vi "recover.vi"(8 "error in (no error)":errorcluster, 11 "Camera Handle":u32=16842752) -> (0 "error out":errorcluster, 2 "Temperature":dbl=-75.0, 3 "Camera Handle":u32=16842752)   [LabVIEW 2015]
uses:
  LabVIEW/Examples2014_6_0_2_9/Fast Examples/Open-Close Hardware/CamHandle.vi
panel:
  out "Pixel Time":i32=500
  in  "Bypass Cooling":bool
  out "Frame Rate":dbl=1203.5142616440007
  out "Vertical Index":u32
  out "Custom Chip Enabled":bool
  out "Vertical Timing":dbl=3.2
  out "Readout Time":dbl=0.8308999999999999
  out "Bit Depth":i32=16
  out "ReadOut Port":i32=2
  out "ADC Offset":i32=-1
  out "ADC Gain":i32=3
  out "ADC Speed":i32=2000
  in  "Error Code(s)":string="Ready"
  in  "Write Tab Control":T1(tab)=enum."ROI"
  in  "Frames to collect (nframe)":u32=1 min=1 step=1
  in  "Exposure":dbl min=0.0 step=0.001 format="%.3f"
  in  "Timing Mode":u32(ring)=3 items=["Free Run/Timed"=1, "External Sync"=3, "Shift per Trigger"=13]
  in  "Trigger Edge":u32(ring)=2 items=["Positive Edge"=1, "Negative Edge"=2]
  in  "Collection Mode":u32(ring)=1 items=["Focus"=1, "N-Frame"=2, "Asynchronous"=3]
  in  "Readut Mode":u16(ring)=1 items=["Full Frame"=1, "Kinetics"=10]
  in  "Temperature 2":dbl=-75.0 format="%.2f"
  in  "Speed":i32=-2 min=-3 step=1
  in  "Gain":i32(ring)=3 items=["Don't Change "=-1, "Low"=1, "Medium"=2, "High"=3]
  in  "Offset":i32=-1 min=-1 step=1
  in  "Readout Port":i32(ring)=2 items=["Don't Change"=-1, "Low Noise"=1, "High capacity"=2]
  in  "Open":u32
  in  "Close":u32
  in  "Shutter State":u16(ring)=3 items=["Always Closed"=1, "Open Each Exposure"=2, "Open at Begining of Acquisition"=3, "Open While Waiting for Trigger"=4]
  in  "Minium Block Size":u32=1
  in  "Number of Minimum Blocks":u32=1
  in  "Number of Clean/Clears cycles":u32
  in  "Number of Strips per Clean":u32=100
  in  "Continous Cleans":bool
  in  "Skip Serial Register Clean":bool=TRUE
  in  "Kinetics Window Height":u32
  in  "Active Y Size":u32=100
  in  "Post Y":u32=8
  in  "Pre Y":u32=8
  in  "Active X Size":u32=1340
  in  "Post X":u32
  in  "Pre X":u32
  in  "Vertical Timing Index":u32
  in  "Enable  Custom Chip":bool
  in  "Logic Output":u16(ring)=3 items=["Not Scan / Not Reading"=1, "Shutter Open"=2, "Not Ready/Busy"=3, "Always Low"=4, "Always High"=8]
  in  "Invert":bool
  out "Y Size ROI":u32=50
  out "X Size ROI":u32=1340
  in  "Y Bin":u32=100 min=1 step=1
  in  "Y End":u32=100 min=1 step=1
  in  "Y Start":u32=1 min=1 step=1
  in  "X Bin":u32=1 min=1 step=1
  in  "X End":u32=1340 min=1 max=100000 step=1
  in  "X Start":u32=1 min=1 step=1
  in  "Camera Number":u32=1
  in  "INI Flag":bool=TRUE
  # "Triggering"
  # "Seconds"
  # "Temperature"
  # "°C"
  # "ADC"
  # "-3 = Slowest speed\n-2 = Fastest speed\n-1 =Default speed or enter speed in kHz"
  # "Shutter"
  # "Shutter Times"
  # "ms"
  # "Cleans / Clears"
  # "Custom Chip and Timing"
  # "Kinetics Timing"
  # "Logic Output"
  # "Region Of Interest"
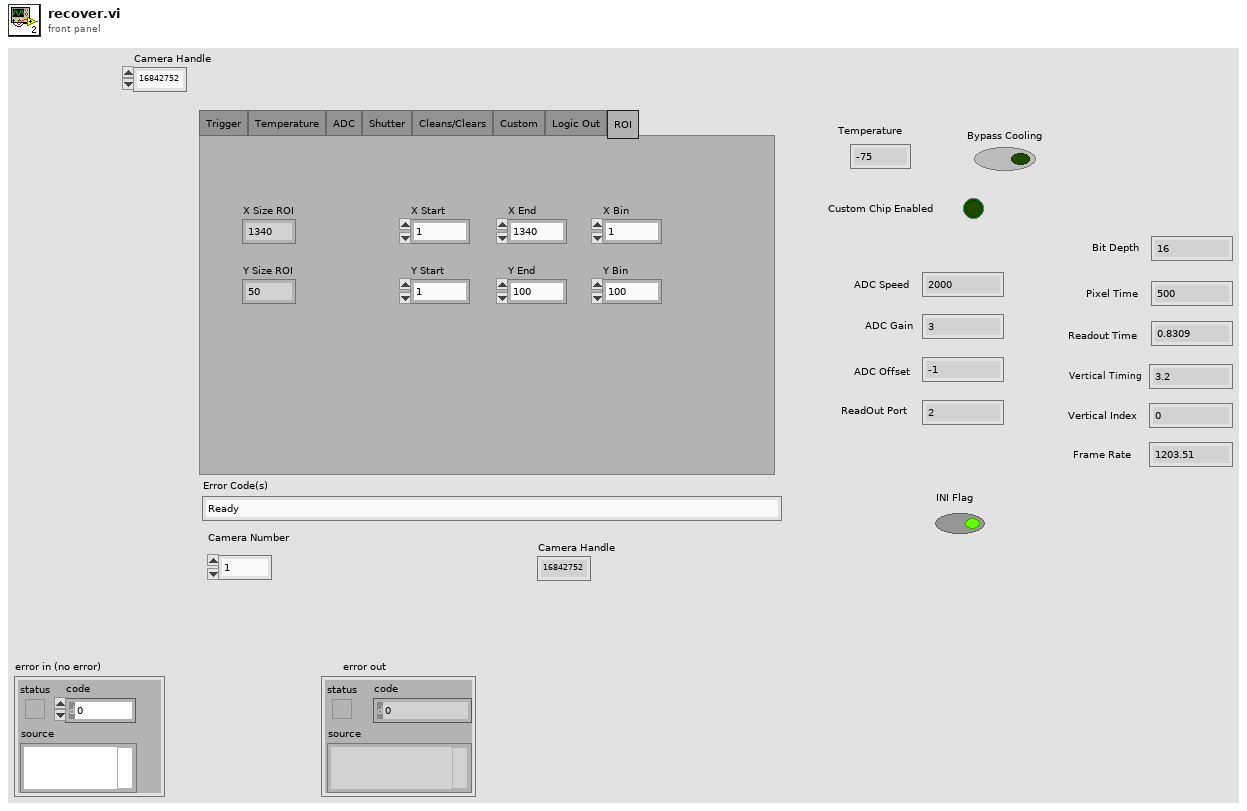
[diagram p1: front panel]
types:
  T1 = enum32{"Trigger", "Temperature", "ADC", "Shutter", "Cleans/Clears", "Custom", "Logic Out", "ROI"}
  T2 = cluster{"Camera Number":i32, "ROI Number":i32, "X Start":i32, "X End":i32, "X Bin":i32, "Y Start":i32, "Y End":i32, "Y Bin":i32}
  T3 = cluster{"Pre Y":u32, "Post Y":u32, "Active Y":u32, "Pre X":u32, "Post X":u32, "Active X":u32, "Custom Chip Enabled":bool, "Vertical Timing Index":u32}
  T4 = cluster{"Exposure":dbl, "Collection Mode":u32, "Timing Mode":u32, "Trigger Edge":u32, "Temperature":dbl}
  T5 = cluster{"ADC Speed":i32, "ADC Gain":i32, "ADC Offset":i32, "Readout Port":i32, "Num Cleans":u32, "Num Strips per Clean":u32, "Mini Block Size":u32, "Num Min Blocks":u32, "Continous Cleans":bool, "Skip Serial Reg Clean":bool}
  T6 = cluster{"Shutter State":u16, "Open Comp Time ":u32, "Close Comp Time":u32, "Logic Out Setting":u32, "Logic Out Invert":bool}
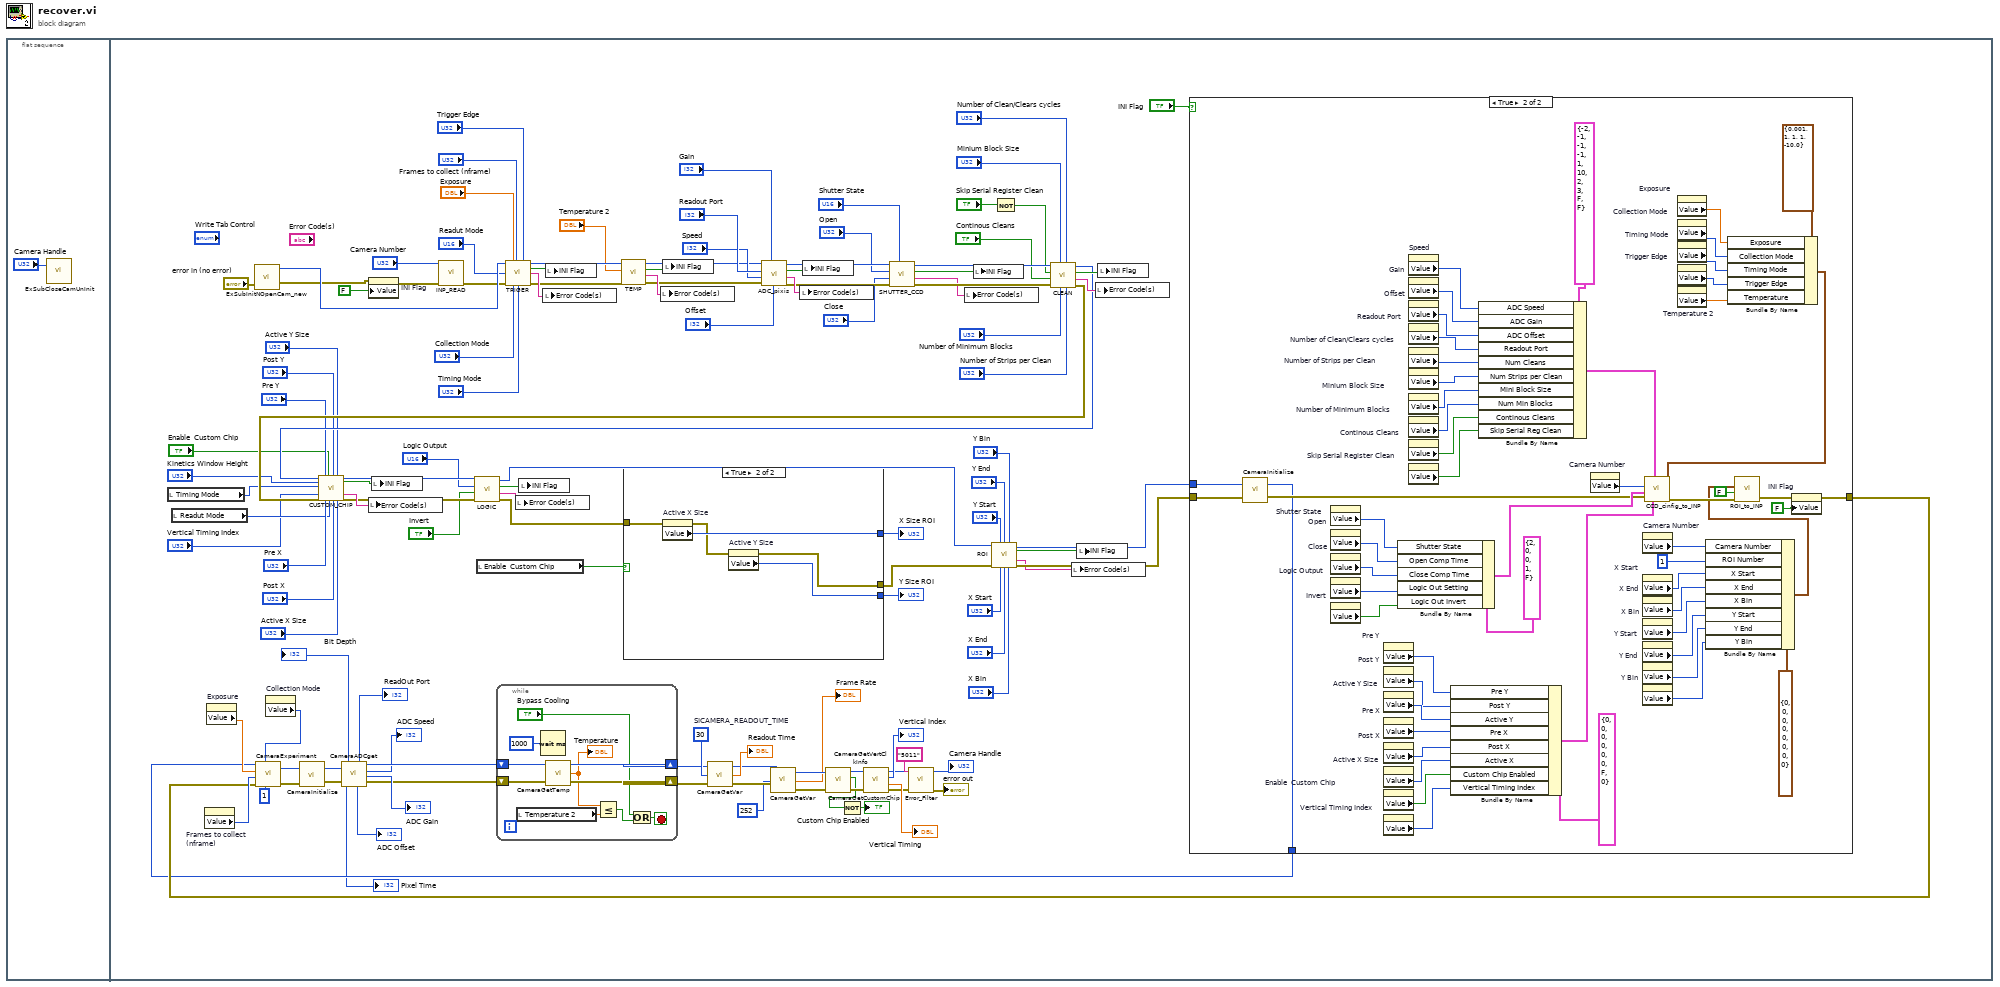
[diagram p0: block diagram]
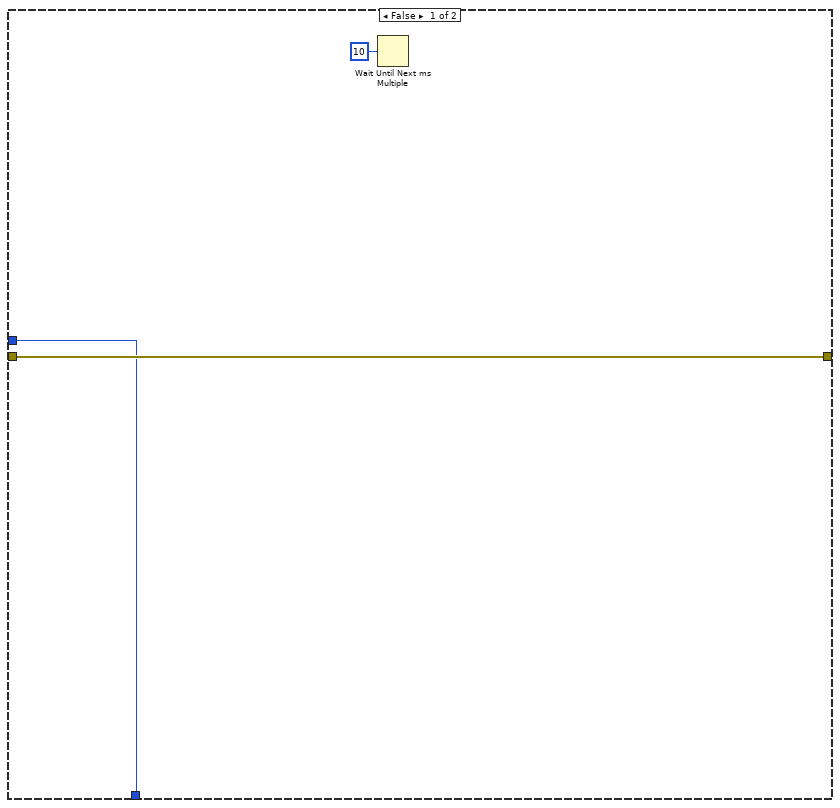
[diagram p2: hidden frame]
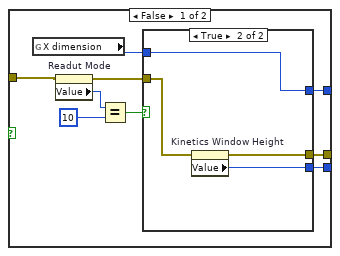
[diagram p3: hidden frame]
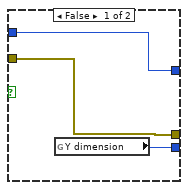
[diagram p4: hidden frame]
diagram:
  n1 = flat-sequence {
    frame #0 {
      n2 = call "ExSubCloseCamUnInit.vi"("Camera Handle"="Camera Handle") -> ()  [unwired: 1 in, 1 out]
    }
    frame #1 {
      w40 = 30  # SICAMERA_READOUT_TIME
      n3 = local read "Timing Mode"() -> (w69:u32)
      n4 = local read "Readut Mode"() -> (w70:u16)
      n5 = property on="Frames to collect (nframe)" class="DigNum (strict)"() -> ("Value"=w19:u32)  [unwired: 2 in, 2 out]
      n6 = property on="Exposure" class="DigNum (strict)"() -> ("Value"=w22:dbl)  [unwired: 2 in, 2 out]
      n7 = call "ExSubInitNOpenCam_new.vi"("error in (no error)"="error in (no error)") -> ("Camera Handle"=w121:u32, "error out"=w6:errorcluster)  [unwired: 1 out]
      n8 = property on="Collection Mode" class="Ring (strict)"() -> ("Value"=w17:u32)  [unwired: 2 in, 2 out]
      n9 = property on="INI Flag" class="Bool (strict)"(error in=w6, "Value"=FALSE) -> (error out=w106:errorcluster)  [unwired: 1 in, 1 out]
      n10 = call "INP_READ.vi"("error in (no error)"=w106, "Camera Number"="Camera Number") -> ("error out"=w105:errorcluster)  [unwired: 4 in, 5 out]
      n11 = local read "Enable  Custom Chip"() -> (w60:bool)
      n12 = call "TRIGER.vi"("Camera Handle"=w121, "Exposure (sec)"="Exposure", "Number of frams"="Frames to collect (nframe)", "Trigger Edge"="Trigger Edge", "ReadOut Mode"="Readut Mode", "error out"=w105, "Acquire / Focus Flag"="Collection Mode", "Timing Mode"="Timing Mode") -> ("Camera Handle"=w112:u32, "INI Flag"=w114:bool, "String"=w113:string, "error out"=w111:errorcluster)  [unwired: 4 in]
      n13 = local write "Error Code(s)"(w113) -> ()
      n14 = local write "INI Flag"(w114) -> ()
      n15 = call "TEMP.vi"("error in (no error)"=w111, "Temperature"="Temperature 2", "Camera Handle"=w112) -> ("error out"=w102:errorcluster, "String"=w109:string, "INI Flag"=w108:bool, "Camera Handle"=w97:u32)  [unwired: 5 in]
      n16 = local write "Error Code(s)"(w109) -> ()
      n17 = local write "INI Flag"(w108) -> ()
      n18 = call "ADC_pixis.vi"("ADC offset"="Offset", "ADC Gain"="Gain", "error in (no error)"=w102, "ADC Speed"="Speed", "Read Out port"="Readout Port", "Camera Handle"=w97) -> ("error out"=w95:errorcluster, "string"=w98:string, "INI Flag"=w99:bool, "Camera Handle"=w96:u32)  [unwired: 2 in]
      n19 = local write "Error Code(s)"(w98) -> ()
      n20 = local write "INI Flag"(w99) -> ()
      n21 = call "SHUTTER_CCD.vi"("Shutter State"="Shutter State", "error out"=w95, "Shutter Comp Time: Pre Open"="Close", "Shutter Comp Time: Post Open"="Open", "Camera Handle"=w96) -> ("error out"=w90:errorcluster, "String"=w89:string, "INI Flag"=w88:bool, "Camera Handle"=w91:u32)  [unwired: 3 in]
      n22 = local write "Error Code(s)"(w89) -> ()
      n23 = local write "INI Flag"(w88) -> ()
      n24 = Not(x="Skip Serial Register Clean") -> (.not. x?=w11:bool)
      n25 = call "CLEAN.vi"("Number of Strips Per Clear"="Number of Strips per Clean", "Number of Clears"="Number of Clean/Clears cycles", "Number of Minimum blocks"="Number of Minimum Blocks", "Minimum Block Size"="Minium Block Size", "error out"=w90, "Continous Clean"="Continous Cleans", "Skip Serial Reg Clean"=w11, "Camera Handle"=w91) -> ("error out 2"=w79:errorcluster, "String"=w82:string, "INI Flag"=w81:bool, "CameraHandle"=w80:u32)
      n26 = call "CUSTOM_CHIP.vi"("Camera Handle"=w80, "Window Size"="Kinetics Window Height", "TriggerMode"=w69, "Vertical Clock"="Vertical Timing Index", "error out"=w79, "Pre Y"="Pre Y", "Pre X"="Pre X", "Enable / Disable Custom Chip"="Enable  Custom Chip", "ReadOut Mode"=w70, "Post Y"="Post Y", "Post X"="Post X", "Parallel (Y) Size"="Active Y Size", "Serial (X) Size"="Active X Size") -> ("Camera Handle"=w66:u32, "INI Flag"=w72:bool, "String"=w71:string, "error out"=w65:errorcluster)  [unwired: 3 in]
      n27 = local write "Error Code(s)"(w71) -> ()
      n28 = local write "INI Flag"(w72) -> ()
      n29 = call "LOGIC.vi"("error out"=w65, "Invert"="Invert", "Logic Output"="Logic Output", "Camera Handle"=w66) -> ("error out 2"=w59:errorcluster, "String"=w61:string, "INI Flag"=w62:bool, "Camera Handle"=w58:u32)  [unwired: 4 in]
      n30 = local write "Error Code(s)"(w61) -> ()
      n31 = local write "INI Flag"(w62) -> ()
      n32 = case shown="True" w60 {
        tunnel: [w197 w213] -> w49
        tunnel: [w196 w212] -> w50
        tunnel: w59 -> [w194 w210]
        tunnel: [w195 w209] -> w57
        frame False {
          n33 = global read "CamHandle.vi" "X dimension"() -> (w198:u32)
          n34 = property on="Readut Mode" class="Ring (strict)"(error in=w194) -> (error out=w193:errorcluster, "Value"=w199:u16)  [unwired: 1 in, 1 out]
          n35 = Equal?(x=w199, y=10) -> (x = y?=w200:bool)
          n36 = case shown="True" w200 {
            tunnel: w198 -> [w204 w208]
            tunnel: [w204 w208] -> w197
            tunnel: [w203 w207] -> w196
            tunnel: [w202 w206] -> w195
            tunnel: w193 -> [w202 w205]
            frame False {
              n37 = global read "CamHandle.vi" "Y dimension"() -> (w203:u32)
            }
            frame True {
              n38 = property on="Kinetics Window Height" class="DigNum (strict)"(error in=w205) -> (error out=w206:errorcluster, "Value"=w207:u32)  [unwired: 1 in, 1 out]
            }
          }
        }
        frame True {
          n39 = property on="Active X Size" class="DigNum (strict)"(error in=w210) -> (error out=w211:errorcluster, "Value"=w213:u32)  [unwired: 1 in, 1 out]
          n40 = property on="Active Y Size" class="DigNum (strict)"(error in=w211) -> (error out=w209:errorcluster, "Value"=w212:u32)  [unwired: 1 in, 1 out]
        }
      }
      "X Size ROI" <- w49
      "Y Size ROI" <- w50
      n41 = call "ROI.vi"("Camera Handle"=w58, "Y Start"="Y Start", "Y End"="Y End", "Y Bin"="Y Bin", "error in"=w57, "X Start"="X Start", "X End"="X End", "X Bin"="X Bin") -> ("Camera Handle"=w16:u32, "INI Flag"=w48:bool, "String"=w7:string, "error out"=w15:errorcluster)  [unwired: 4 in]
      n42 = local write "Error Code(s)"(w7) -> ()
      n43 = local write "INI Flag"(w48) -> ()
      n44 = local write "Error Code(s)"(w82) -> ()
      n45 = local write "INI Flag"(w81) -> ()
      n46 = case shown="True" "INI Flag" {
        tunnel: w15 -> [w136 w164]
        tunnel: [w136 w162] -> w5
        tunnel: w16 -> [w134 w138]
        tunnel: [w134 w137] -> w4
        frame False {
          n47 = Wait Until Next ms Multiple(millisecond multiple=u32 10) -> ()  [unwired: 1 out]
        }
        frame True {
          n48 = call <userlib>:"CameraInitialize.vi"("error in"=w164, "Camera Handle"=w138) -> ("error out"=w165:errorcluster, "Camera Handle"=w137:u32)
          n49 = property on="Shutter State" class="Ring (strict)"() -> ("Value"=w186:u16)  [unwired: 2 in, 2 out]
          n50 = property on="Open" class="DigNum (strict)"() -> ("Value"=w187:u32)  [unwired: 2 in, 2 out]
          n51 = property on="Close" class="DigNum (strict)"() -> ("Value"=w188:u32)  [unwired: 2 in, 2 out]
          n52 = property on="Logic Output" class="Ring (strict)"() -> ("Value"=w189:u16)  [unwired: 2 in, 2 out]
          n53 = property on="Invert" class="Bool (strict)"() -> ("Value"=w190:bool)  [unwired: 2 in, 2 out]
          n54 = property on="Pre Y" class="DigNum (strict)"() -> ("Value"=w159:u32)  [unwired: 2 in, 2 out]
          n55 = property on="Post Y" class="DigNum (strict)"() -> ("Value"=w151:u32)  [unwired: 2 in, 2 out]
          n56 = property on="Active Y Size" class="DigNum (strict)"() -> ("Value"=w154:u32)  [unwired: 2 in, 2 out]
          n57 = property on="Pre X" class="DigNum (strict)"() -> ("Value"=w158:u32)  [unwired: 2 in, 2 out]
          n58 = property on="Post X" class="DigNum (strict)"() -> ("Value"=w152:u32)  [unwired: 2 in, 2 out]
          n59 = property on="Active X Size" class="DigNum (strict)"() -> ("Value"=w157:u32)  [unwired: 2 in, 2 out]
          n60 = property on="Enable  Custom Chip" class="Bool (strict)"() -> ("Value"=w156:bool)  [unwired: 2 in, 2 out]
          n61 = property on="Vertical Timing Index" class="DigNum (strict)"() -> ("Value"=w155:u32)  [unwired: 2 in, 2 out]
          n62 = Bundle By Name(cluster=T6 {"Shutter State"=2, "Open Comp Time "=0, "Close Comp Time"=0, "Logic Out Setting"=1, "Logic Out Invert"=FALSE} ("Shutter and Logic Out"), "Shutter State"=w186, "Open Comp Time"=w187, "Close Comp Time"=w188, "Logic Out Setting"=w189, "Logic Out Invert"=w190) -> (w191:T6)
          n63 = property on="Speed" class="DigNum (strict)"() -> ("Value"=w183:i32)  [unwired: 2 in, 2 out]
          n64 = property on="Gain" class="Ring (strict)"() -> ("Value"=w182:i32)  [unwired: 2 in, 2 out]
          n65 = property on="Offset" class="DigNum (strict)"() -> ("Value"=w180:i32)  [unwired: 2 in, 2 out]
          n66 = property on="Readout Port" class="Ring (strict)"() -> ("Value"=w178:i32)  [unwired: 2 in, 2 out]
          n67 = property on="Number of Clean/Clears cycles" class="DigNum (strict)"() -> ("Value"=w177:u32)  [unwired: 2 in, 2 out]
          n68 = property on="Number of Strips per Clean" class="DigNum (strict)"() -> ("Value"=w176:u32)  [unwired: 2 in, 2 out]
          n69 = property on="Minium Block Size" class="DigNum (strict)"() -> ("Value"=w174:u32)  [unwired: 2 in, 2 out]
          n70 = property on="Number of Minimum Blocks" class="DigNum (strict)"() -> ("Value"=w175:u32)  [unwired: 2 in, 2 out]
          n71 = property on="Continous Cleans" class="Bool (strict)"() -> ("Value"=w179:bool)  [unwired: 2 in, 2 out]
          n72 = property on="Skip Serial Register Clean" class="Bool (strict)"() -> ("Value"=w181:bool)  [unwired: 2 in, 2 out]
          n73 = Bundle By Name(cluster=T3 {"Pre Y"=0, "Post Y"=0, "Active Y"=0, "Pre X"=0, "Post X"=0, "Active X"=0, "Custom Chip Enabled"=FALSE, "Vertical Timing Index"=0} ("Custom Chip"), "Pre Y"=w159, "Post Y"=w151, "Active Y"=w154, "Pre X"=w158, "Post X"=w152, "Active X"=w157, "Custom Chip Enabled"=w156, "Vertical Timing Index"=w155) -> (w153:T3)
          n74 = Bundle By Name(cluster=T5 {"ADC Speed"=-2, "ADC Gain"=-1, "ADC Offset"=-1, "Readout Port"=-1, "Num Cleans"=1, "Num Strips per Clean"=10, "Mini Block Size"=2, "Num Min Blocks"=3, "Continous Cleans"=FALSE, "Skip Serial Reg Clean"=FALSE} ("ADC and Cleans"), "ADC Speed"=w183, "ADC Gain"=w182, "ADC Offset"=w180, "Readout Port"=w178, "Num Cleans"=w177, "Num Strips per Clean"=w176, "Mini Block Size"=w174, "Num Min Blocks"=w175, "Continous Cleans"=w179, "Skip Serial Reg Clean"=w181) -> (w184:T5)
          n75 = property on="Camera Number" class="DigNum (strict)"() -> ("Value"=w166:u32)  [unwired: 2 in, 2 out]
          n76 = property on="Camera Number" class="DigNum (strict)"() -> ("Value"=w148:u32)  [unwired: 2 in, 2 out]
          n77 = property on="X Start" class="DigNum (strict)"() -> ("Value"=w146:u32)  [unwired: 2 in, 2 out]
          n78 = property on="X End" class="DigNum (strict)"() -> ("Value"=w145:u32)  [unwired: 2 in, 2 out]
          n79 = property on="X Bin" class="DigNum (strict)"() -> ("Value"=w144:u32)  [unwired: 2 in, 2 out]
          n80 = property on="Y Start" class="DigNum (strict)"() -> ("Value"=w143:u32)  [unwired: 2 in, 2 out]
          n81 = property on="Y End" class="DigNum (strict)"() -> ("Value"=w142:u32)  [unwired: 2 in, 2 out]
          n82 = property on="Y Bin" class="DigNum (strict)"() -> ("Value"=w141:u32)  [unwired: 2 in, 2 out]
          n83 = property on="Exposure" class="DigNum (strict)"() -> ("Value"=w167:dbl)  [unwired: 2 in, 2 out]
          n84 = property on="Collection Mode" class="Ring (strict)"() -> ("Value"=w168:u32)  [unwired: 2 in, 2 out]
          n85 = property on="Timing Mode" class="Ring (strict)"() -> ("Value"=w169:u32)  [unwired: 2 in, 2 out]
          n86 = property on="Trigger Edge" class="Ring (strict)"() -> ("Value"=w170:u32)  [unwired: 2 in, 2 out]
          n87 = property on="Temperature 2" class="DigNum (strict)"() -> ("Value"=w171:dbl)  [unwired: 2 in, 2 out]
          n88 = Bundle By Name(cluster=T2 {"Camera Number"=0, "ROI Number"=0, "X Start"=0, "X End"=0, "X Bin"=0, "Y Start"=0, "Y End"=0, "Y Bin"=0} ("ROI Values"), "Camera Number"=w148, "ROI Number"=1, "X Start"=w146, "X End"=w145, "X Bin"=w144, "Y Start"=w143, "Y End"=w142, "Y Bin"=w141) -> (w140:T2)
          n89 = Bundle By Name(cluster=T4 {"Exposure"=0.001, "Collection Mode"=1, "Timing Mode"=1, "Trigger Edge"=1, "Temperature"=-10.0} ("Timing and Temperature"), "Exposure"=w167, "Collection Mode"=w168, "Timing Mode"=w169, "Trigger Edge"=w170, "Temperature"=w171) -> (w172:T4)
          n90 = call "CCD_cinfig_to_INP.vi"("Timing and Temperature"=w172, "Custom Chip"=w153, "ADC and Cleans"=w184, "error in (no error)"=w165, "Shutter and Logic Out"=w191, "Camera Number"=w166) -> ("error out"=w163:errorcluster)  [unwired: 5 in]
          n91 = call "ROI_to_INP.vi"("error in (no error)"=w163, "Show Message"=FALSE, "ROI Values"=w140) -> ("error out"=w150:errorcluster)  [unwired: 8 in]
          n92 = property on="INI Flag" class="Bool (strict)"(error in=w150, "Value"=FALSE) -> (error out=w162:errorcluster)  [unwired: 1 in, 1 out]
        }
      }
      n93 = call <userlib>:"CameraExperiment.vi"("Number of Accumulations"=1, "Acquire / Focus Flag"=w17, "error in"=w5, "Number of Images"=w19, "Exposure (sec)"=w22, "Camera Handle"=w4) -> ("error out"=w24:errorcluster, "Camera Handle"=w23:u32)
      n94 = call <userlib>:"CameraInitialize.vi"("error in"=w24, "Camera Handle"=w23) -> ("error out"=w26:errorcluster, "Camera Handle"=w25:u32)
      n95 = call <userlib>:"CameraADCget.vi"("Camera handle"=w25, "error in (no error)"=w26) -> ("Bit Depth"=→"Bit Depth":i32, "Pixel Time"=→"Pixel Time":i32, "Readout Port"=→"ReadOut Port":i32, "ADC Offset"=→"ADC Offset":i32, "Camera handle"=w41:u32, "ADC Speed"=→"ADC Speed":i32, "ADC Gain"=→"ADC Gain":i32, "error out"=w42:errorcluster)
      n96 = while {
        shift-right: [w131] -> w39
        shift-left: w42 -> [w133]
        shift-right: [w130] -> w38
        shift-left: w41 -> [w132]
        stop <- w126 stop-if-true
        n97 = local read "Temperature 2"() -> (w128:dbl)
        n98 = Wait (ms)(milliseconds to wait=u32 1000) -> ()  [unwired: 1 out]
        n99 = call <userlib>:"CameraGetTemp.vi"("Camera Handle"=w132, "error in (no error)"=w133) -> ("Camera Handle"=w130:u32, "Temperature"=w129:dbl, "error out"=w131:errorcluster)
        "Temperature" <- w129
        n100 = Less Or Equal?(x=w129, y=w128) -> (x <= y?=w124:bool)
        n101 = Or(x="Bypass Cooling", y=w124) -> (x .or. y?=w126:bool)
      }
      n102 = call <userlib>:"CameraGetVar.vi"("error in"=w39, "Parameter ID"=w40, "Camera Handle"=w38) -> ("error out"=w32:errorcluster, "Value"=→"Readout Time":dbl, "Camera Handle"=w30:u32)
      n103 = call <userlib>:"CameraGetVar.vi"("error in"=w32, "Parameter ID"=252, "Camera Handle"=w30) -> ("error out"=w31:errorcluster, "Value"=→"Frame Rate":dbl, "Camera Handle"=w29:u32)
      n104 = call <userlib>:"CameraGetCustomChip.vi"("Camera Handle"=w29, "error in (no error)"=w31) -> ("Camera Handle"=w36:u32, "Custum chip Enable/Disable status"=w9:bool, "error out"=w35:errorcluster)  [unwired: 1 out]
      n105 = Not(x=w9) -> (.not. x?=→"Custom Chip Enabled":bool)
      n106 = call <userlib>:"CameraGetVertClkInfo.vi"("Camera Handle"=w36, "error in (no error)"=w35) -> ("Camera Handle"=→"Camera Handle":u32, "VertClk index"=→"Vertical Index":u32, "Real Clock Value"=→"Vertical Timing":dbl, "error out"=w21:errorcluster)  [unwired: 2 out]
      n107 = call "Error_Filter.vi"("error in (no error)"=w21, "Error Numbers To Filter"="5011") -> ("error out"=→"error out":errorcluster)  [unwired: 9 in]
    }
  }
